vi "Get Stimulus Fit.vi"(8 "error in (no error)":errorcluster, 11 "Abstract Fit in":refnum<class "Abstract Fit.lvclass">) -> (0 "error out":errorcluster, 2 "Fit out":dbl[](array[numeric]), 3 "Abstract Fit out":refnum<class "Abstract Fit.lvclass">)   [LabVIEW 2013, in "Abstract Fit.lvclass"]
uses:
  Abstract Fit.lvclass
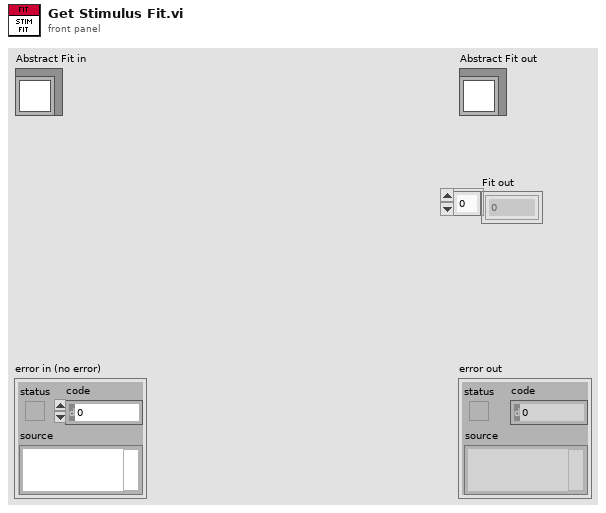
[diagram p1: front panel]
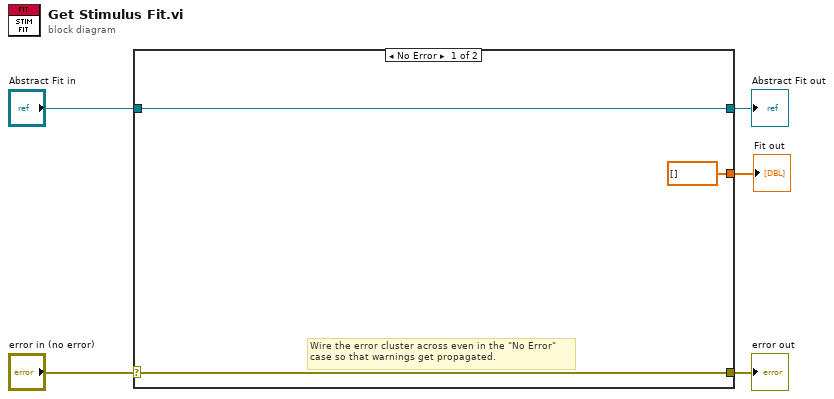
[diagram p0: block diagram]
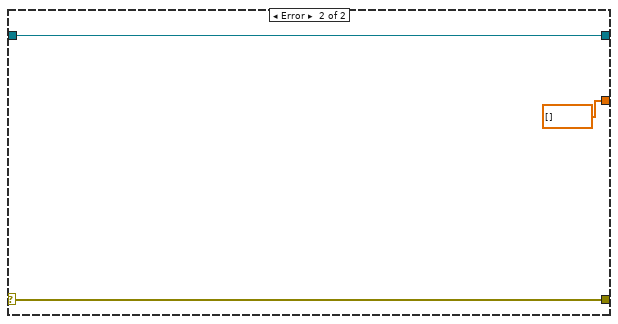
[diagram p2: hidden frame]
diagram:
  n1 = case shown="No Error" "error in (no error)" {
    selector: "error in (no error)" -> [w8 w11]
    tunnel: [w8 w11] -> w4
    tunnel: [w7 w10] -> w2
    tunnel: "Abstract Fit in" -> [w7 w10]
    tunnel: [dbl[] [] ("Y") dbl[] [] ("Y")] -> w1
    frame No Error {
      # "Wire the error cluster across even in the \"No Error\"\ncase so that warnings get propagated."
    }
    frame Error {
    }
  }
  "error out" <- w4
  "Abstract Fit out" <- w2
  "Fit out" <- w1
